vi "AB_Engine_Construct_PPL_Table.vi"(8 "error in (no error)":errorcluster, 11 "sources in":refnum<class "AB_Source.lvclass">[](array[class])) -> (0 "error out":errorcluster, 2 "PPL Table":variant, 3 "sources out":refnum<class "AB_Source.lvclass">[](array[class]))   [LabVIEW 2020]
uses:
  <vilib>/AppBuilder/AB_Classes/Source/AB_Source.lvclass
  <vilib>/AppBuilder/Engine/AB_Engine_PPL_Source_Index.ctl
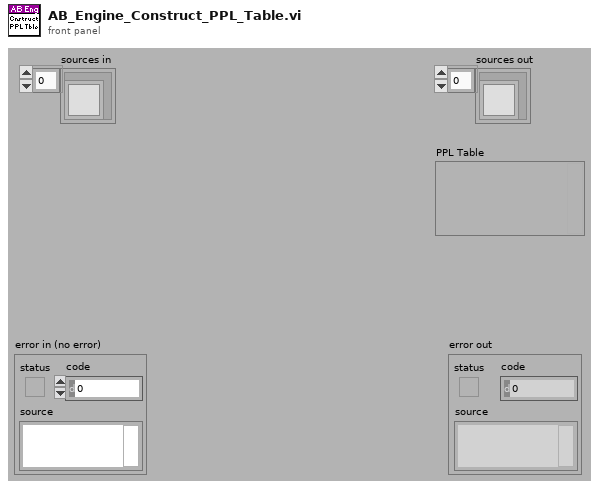
[diagram p1: front panel]
types:
  T1 = typedef "AB_Engine_PPL_Source_Index.ctl" = cluster{"path":path, "source index":i32, "PPL?":bool}
  T2 = typedef "AB_Source.ctl" = cluster{"path":path, "itemID":string, "parentIndex":i32, "sourceInclusion":T3, "destinationIndex":i32, "properties":T4[], "newName":string, "lvfile":bool, "valid":bool, "eng_inBuild":bool, "eng_isNonVILink":bool, "Amalgamation":bool, "Amalgamation Piece":bool, "eng_delimitedName":string, "preventRename":bool}
  T3 = typedef "AB_Source_Inclusion.ctl" = enum16{"IncludeIfReferenced", "Include", "Exclude", "TopLevel"}
  T4 = typedef "AB_Source_Properties.ctl" = cluster{"sourcePropertyType":T5, "value":variant}
  T5 = typedef "AB_Source_Property_Type.ctl" = enum16{"Remove block diagram", "Remove front panel", "Password", "Window has title bar", "Show menu bar", "Show vertical scroll bar", "Show horizontal scroll bar", "Show toolbar", "Show Abort button", "Show fp when called", "Window behavior", "Allow user to close window", "Window run-time position", "Run when opened", "Allow debugging", "Auto error handling", "Generate guard code", "Use stack variables", "Expression folding", "Integer only", "Inline subVI"}
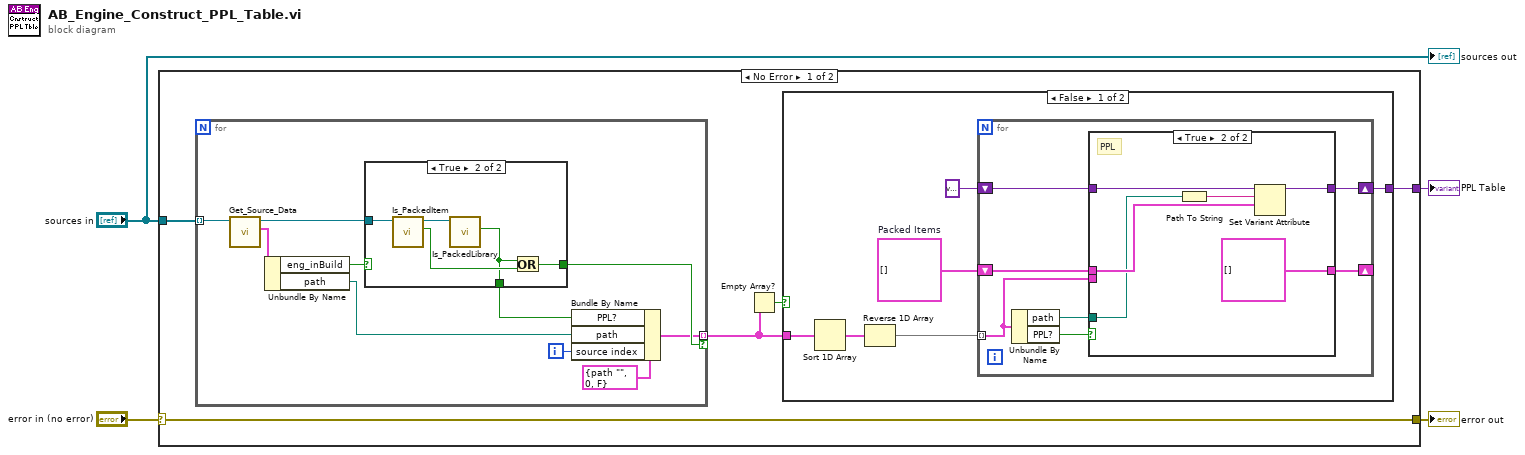
[diagram p0: block diagram]
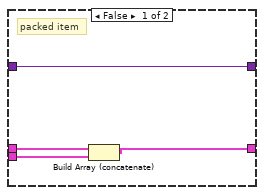
[diagram p2: hidden frame]
diagram:
  n1 = case shown="No Error" "error in (no error)" {
    selector: "error in (no error)" -> [w8 w48]
    tunnel: [w8 w48] -> w3
    tunnel: "sources in" -> [w9 _]
    tunnel: [w5 _] -> w1
    frame No Error {
      n2 = for {
        tunnel: w9 -> [w41] mode=indexing
        tunnel: [w33] -> w6 mode=indexing if=w42
        i -> [w35]
        n3 = call <vilib>:"Get_Source_Data.vi"("Class in"=w41) -> ("data"=w39:T2, "Class out"=w40:refnum<class "AB_Source.lvclass">)  [unwired: 8 in, 1 out]
        n4 = Unbundle By Name(w39) -> ("eng_inBuild"=w38:bool, "path"=w36:path)
        n5 = case shown="True" w38 {
          tunnel: [_ w45] -> w42
          tunnel: w40 -> [_ w44]
          tunnel: [_ w43] -> w34
          frame False {
          }
          frame True {
            n6 = call-dynamic "Is_PackedItem.vi"("AB_Source in"=w44) -> ("packed item"=w46:bool, "AB_Source out"=w47:refnum<class "AB_Source.lvclass">)  [unwired: 8 in, 1 out]
            n7 = call <vilib>:"Is_PackedLibrary.vi"("AB_Source in"=w47) -> ("PPL?"=w43:bool)  [unwired: 7 in, 3 out]
            n8 = Or(x=w43, y=w46) -> (x .or. y?=w45:bool)
          }
        }
        n9 = Bundle By Name(cluster=T1 {"path"=path "", "source index"=0, "PPL?"=FALSE} ("output cluster"), "PPL?"=w34, "path"=w36, "source index"=w35) -> (w33:T1)
      }
      n10 = Empty Array?(array=w6) -> (empty?=w7:bool)
      n11 = case shown="False" w7 {
        tunnel: w6 -> [w15 _]
        tunnel: [w11 _] -> w5
        frame False {
          w12 = T1[] []  # Packed Items
          n12 = Sort 1D Array(array=w15) -> (sorted array=w14:T1[])
          n13 = Reverse 1D Array(array=w14) -> (reversed array=w13:T1[])
          n14 = for {
            tunnel: w13 -> [w20] mode=indexing
            shift-right: [w19] -> w11
            shift-left: variant -> [w21]
            shift-right: [w17] -> _
            shift-left: w12 -> [w18]
            n15 = Unbundle By Name(w20) -> ("path"=w16:path, "PPL?"=w22:bool)
            n16 = case shown="True" w22 {
              tunnel: w21 -> [w26 w31]
              tunnel: w20 -> [w24 _]
              tunnel: [w26 w30] -> w19
              tunnel: w18 -> [w25 w29]
              tunnel: [w23 T1[] []] -> w17
              tunnel: w16 -> [_ w28]
              frame False {
                # "packed item"
                n17 = Build Array (concatenate)(w25, w24) -> (w23:T1[])
              }
              frame True {
                # "PPL"
                n18 = Path To String(path=w28) -> (string=w27:string)
                n19 = Set Variant Attribute(Variant=w31, name=w27, value=w29) -> (Variant out=w30:variant)  [unwired: 1 in, 2 out]
              }
            }
          }
        }
        frame True {
        }
      }
    }
    frame Error {
    }
  }
  "error out" <- w3
  "PPL Table" <- w1
  "sources out" <- "sources in"
